vi "Tree Expand.vi"(0 "Tree Reference In":refnum<vi>, 5 "error in (no error)":errorcluster) -> (14 "Tree Reference Out":refnum<vi>, 19 "error out":errorcluster)   [LabVIEW 2014]
doc: "Expands the entire tree"
panel:
  # "VI INPUTS"
  # "VI OUTPUTS"
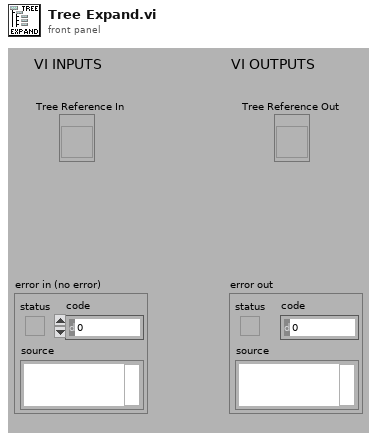
[diagram p1: front panel]
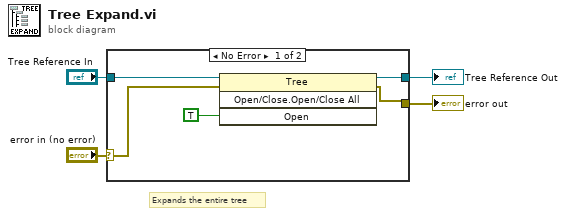
[diagram p0: block diagram]
diagram:
  # "Expands the entire tree"
  n1 = case shown="No Error" "error in (no error)" {
    selector: "error in (no error)" -> [w6 w10]
    tunnel: "Tree Reference In" -> [w7 w11]
    tunnel: [w9 w11] -> w3
    tunnel: [w8 w10] -> w2
    frame No Error {
      n2 = invoke class="Tree" method="Open/Close.Open/Close All"(reference=w7, error in=w6, "Open"=TRUE ("Delete Children")) -> (reference out=w9:refnum<vi>, error out=w8:errorcluster)  [unwired: 1 in, 2 out]
    }
    frame Error {
    }
  }
  "Tree Reference Out" <- w3
  "error out" <- w2
